vi "Load Cell.vi"() -> ()   [LabVIEW 2018]
uses:
  <vilib>/ptbypt/NI_PtbyPt.lvlib
  <vilib>/Analysis/NI_AALPro.lvlib
panel:
  out "Measured Voltage - V":dbl
  in  "sample length for \nmoving average":i32(slide)=100 scale=0.0..10.0
  in  "stop":bool
  out "Raw Voltage Chart":dbl(graph)
  out "Weight, N":dbl
  out "Output Std Dev, V":dbl
  out "Input Std Dev, N":dbl
  out "Slope, V/N":dbl
  out "Intercept, V":dbl
  out "Calibration Graph":cluster{dbl[], "Best Linear Fit":dbl[]}[](graph)
  out "Measurement Chart":cluster{dbl, "mean":dbl}(graph)
  in  "Take Data Points":bool caption="Take Data Point"
  in  "Mass - g":dbl
  in  "Real Data":bool
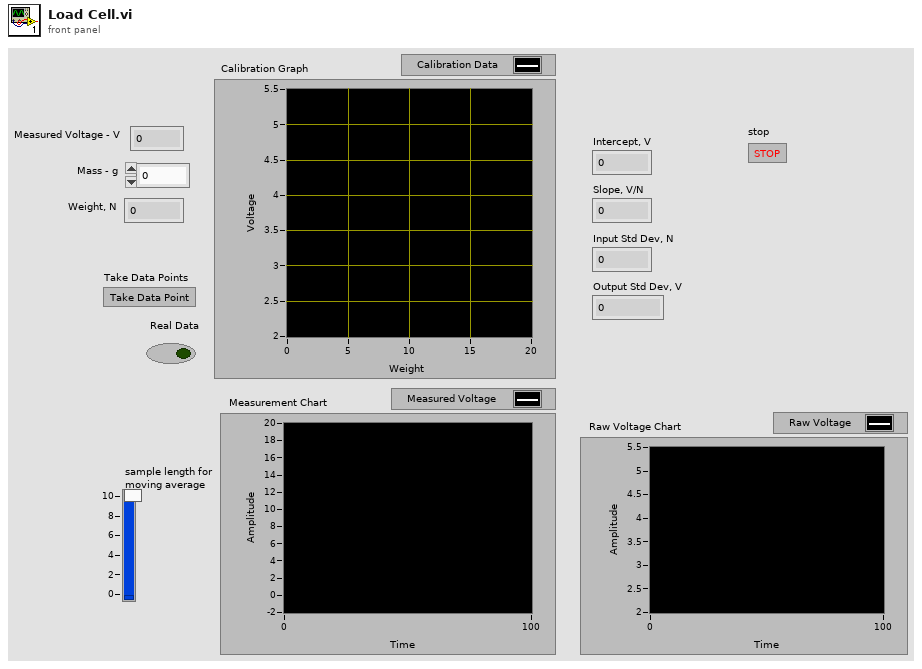
[diagram p1: front panel]
types:
  T1 = cluster{"Array":dbl[], "Best Linear Fit":dbl[]}[]
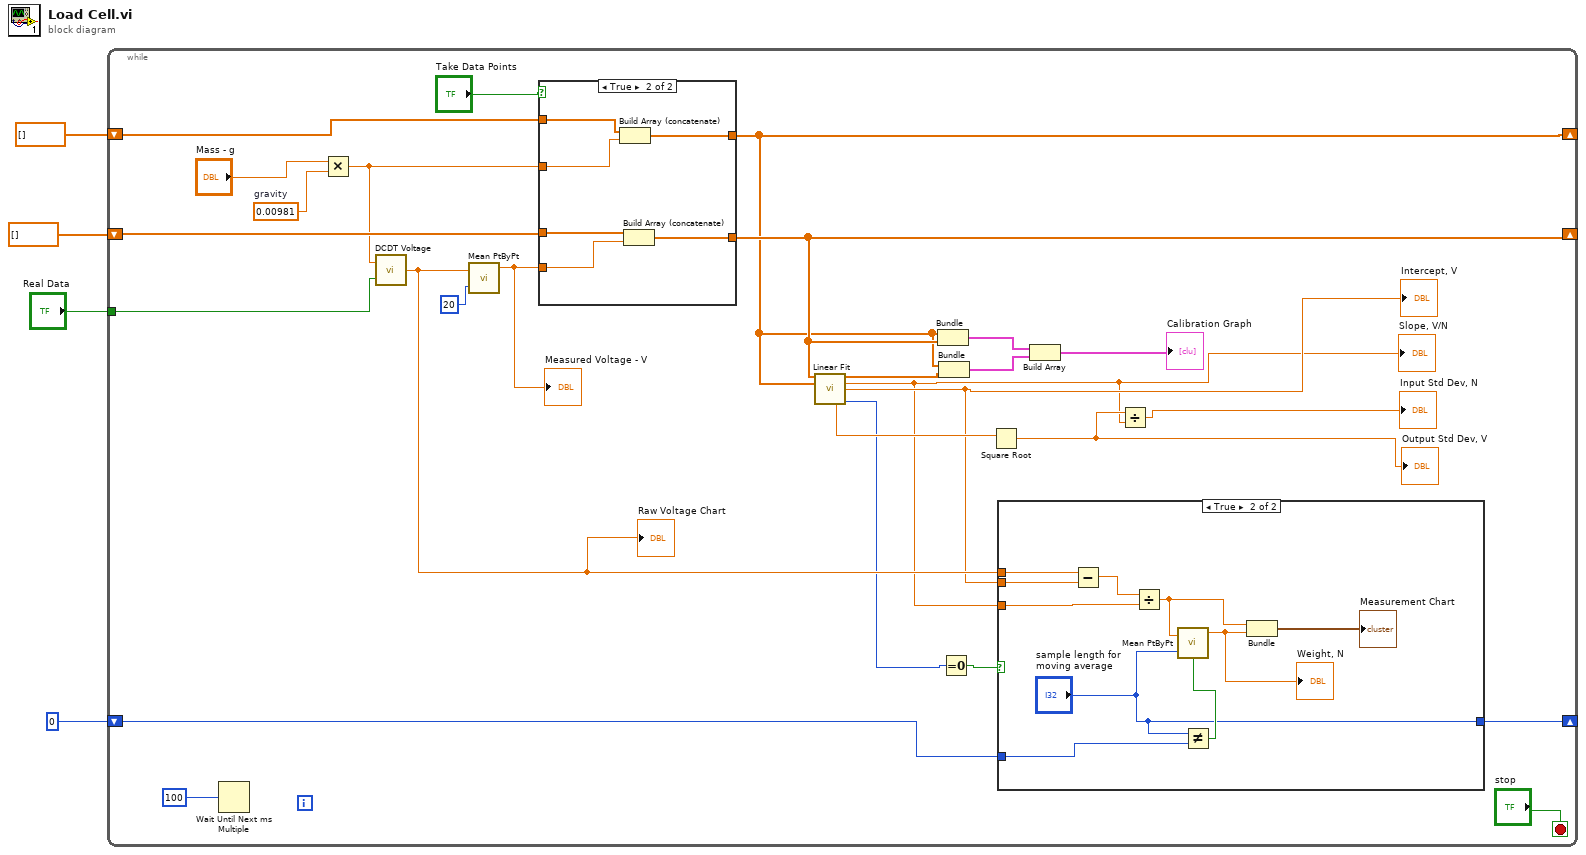
[diagram p0: block diagram]
diagram:
  n1 = while {
    shift-right: [w29] -> _
    shift-left: 0 -> [w25]
    tunnel: "Real Data" -> [w7]
    shift-right: [w11] -> _
    shift-left: dbl[] [] ("Array") -> [w26]
    shift-right: [w10] -> _
    shift-left: dbl[] [] ("Array") -> [w27]
    stop <- "stop" stop-if-true
    w28 = 0.00981  # gravity
    n2 = Wait Until Next ms Multiple(millisecond multiple=100) -> ()  [unwired: 1 out]
    n3 = Multiply(x="Mass - g", y=w28) -> (x*y=w6:dbl)
    n4 = call "DCDT Voltage.vi"("Real Data"=w7, "Weight"=w6) -> ("Voltage"=w15:dbl)
    "Raw Voltage Chart" <- w15
    n5 = call <vilib>:"Mean PtByPt.vi"("x"=w15, "sample length"=20) -> ("mean"=w5:dbl)  [unwired: 2 in, 1 out]
    "Measured Voltage - V" <- w5
    n6 = case shown="True" "Take Data Points" {
      tunnel: w6 -> [_ w50]
      tunnel: w27 -> [w44 w49]
      tunnel: w26 -> [w43 w48]
      tunnel: w5 -> [_ w47]
      tunnel: [w44 w46] -> w10
      tunnel: [w43 w45] -> w11
      frame False {
      }
      frame True {
        n7 = Build Array (concatenate)(w49, w50) -> (w46:dbl[])
        n8 = Build Array (concatenate)(w48, w47) -> (w45:dbl[])
      }
    }
    n9 = call <vilib>:"Linear Fit.vi"("Y"=w11, "X"=w10) -> ("Best Linear Fit"=w23:dbl[], "slope"=w8:dbl, "intercept"=w9:dbl, "residue"=w18:dbl, "error"=w13:i32)  [unwired: 9 in]
    "Slope, V/N" <- w8
    "Intercept, V" <- w9
    n10 = Bundle("Array"=w10, "Array"=w11) -> (w22:cluster{"Array":dbl[], "Array":dbl[]})  [unwired: 1 in]
    n11 = Bundle("Array"=w10, "Best Linear Fit"=w23) -> (w21:cluster{"Array":dbl[], "Best Linear Fit":dbl[]})  [unwired: 1 in]
    n12 = Equal To 0?(x=w13) -> (x = 0?=w12:bool)
    n13 = Square Root(x=w18) -> (sqrt(x)=w17:dbl)
    "Output Std Dev, V" <- w17
    n14 = case shown="True" w12 {
      tunnel: w25 -> [w32 w39]
      tunnel: [w32 "sample length for \nmoving average"] -> w29
      tunnel: w15 -> [_ w38]
      tunnel: w8 -> [_ w37]
      tunnel: w9 -> [_ w36]
      frame False {
      }
      frame True {
        n15 = Subtract(x=w38, y=w36) -> (x-y=w42:dbl)
        n16 = Divide(x=w42, y=w37) -> (x/y=w41:dbl)
        n17 = Not Equal?(x="sample length for \nmoving average", y=w39) -> (x != y?=w34:bool)
        n18 = call <vilib>:"Mean PtByPt.vi"("x"=w41, "sample length"="sample length for \nmoving average", "initialize"=w34) -> ("mean"=w35:dbl)  [unwired: 1 in, 1 out]
        "Weight, N" <- w35
        n19 = Bundle(w41, "mean"=w35) -> (→"Measurement Chart":cluster{dbl, "mean":dbl})  [unwired: 1 in]
      }
    }
    n20 = Build Array(w22, w21) -> (→"Calibration Graph":T1)
    n21 = Divide(x=w17, y=w8) -> (x/y=→"Input Std Dev, N":dbl)
  }
